vi "Modbus Test Setup.vi"(6 "Mannequin Data":u16[](array[numeric]), 8 "error in (no error)":errorcluster, 10 "Select test case":i32(listbox), 11 "Queue in":refnum<queue>) -> (0 "error out":errorcluster, 3 "Queue out":refnum<queue>)   [LabVIEW 2023]
uses:
  Message Queue/Message Cluster.ctl
  Message Queue/Enqueue Message (Single).vi
  Message Queue/Message Queue.lvlib
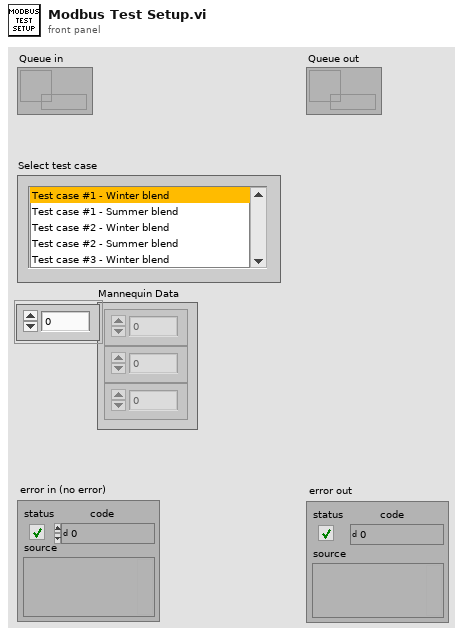
[diagram p1: front panel]
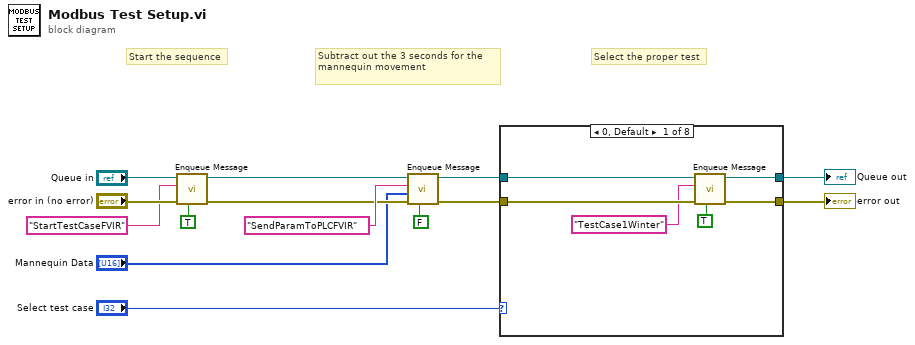
[diagram p0: block diagram]
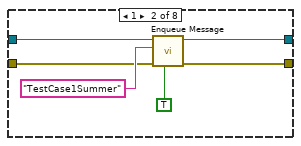
[diagram p2: hidden frame]
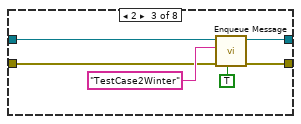
[diagram p3: hidden frame]
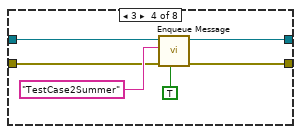
[diagram p4: hidden frame]
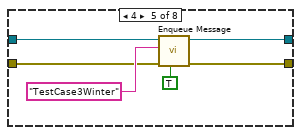
[diagram p5: hidden frame]
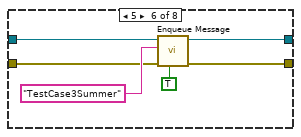
[diagram p6: hidden frame]
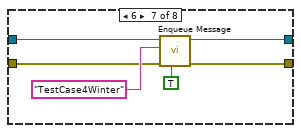
[diagram p7: hidden frame]
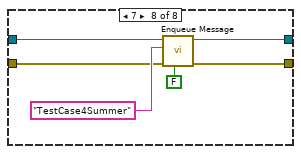
[diagram p8: hidden frame]
diagram:
  # "Select the proper test"
  # "Start the sequence"
  # "Subtract out the 3 seconds for the \nmannequin movement"
  n1 = call-poly "Enqueue Message.vi"("Priority Message? (F)"=TRUE, "error in (no error)"="error in (no error)", "Message"="StartTestCaseFVIR", "Message Queue"="Queue in") -> ("error out"=w2:errorcluster, "dup Message Queue"=w5:refnum<queue>)  [unwired: 6 in]
  n2 = call-poly "Enqueue Message.vi"("Priority Message? (F)"=FALSE, "error in (no error)"=w2, "Message Data"="Mannequin Data", "Message"="SendParamToPLCFVIR", "Message Queue"=w5) -> ("error out"=w3:errorcluster, "dup Message Queue"=w4:refnum<queue>)  [unwired: 5 in]
  n3 = case shown="0, Default" "Select test case" {
    tunnel: w4 -> [w20 w25 w31 w37 w43 w50 w55 w61]
    tunnel: [w17 w24 w30 w36 w42 w49 w54 w60] -> w9
    tunnel: [w19 w23 w29 w35 w41 w48 w53 w59] -> w8
    tunnel: w3 -> [w18 w21 w27 w33 w39 w45 w51 w57]
    frame 0, Default {
      n4 = call-poly "Enqueue Message.vi"("Priority Message? (F)"=TRUE, "error in (no error)"=w18, "Message"="TestCase1Winter", "Message Queue"=w20) -> ("error out"=w17:errorcluster, "dup Message Queue"=w19:refnum<queue>)  [unwired: 6 in]
    }
    frame 1 {
      n5 = call-poly "Enqueue Message.vi"("Priority Message? (F)"=TRUE, "error in (no error)"=w21, "Message"="TestCase1Summer", "Message Queue"=w25) -> ("error out"=w24:errorcluster, "dup Message Queue"=w23:refnum<queue>)  [unwired: 6 in]
    }
    frame 2 {
      n6 = call-poly "Enqueue Message.vi"("Priority Message? (F)"=TRUE, "error in (no error)"=w27, "Message"="TestCase2Winter", "Message Queue"=w31) -> ("error out"=w30:errorcluster, "dup Message Queue"=w29:refnum<queue>)  [unwired: 6 in]
    }
    frame 3 {
      n7 = call-poly "Enqueue Message.vi"("Priority Message? (F)"=TRUE, "error in (no error)"=w33, "Message"="TestCase2Summer", "Message Queue"=w37) -> ("error out"=w36:errorcluster, "dup Message Queue"=w35:refnum<queue>)  [unwired: 6 in]
    }
    frame 4 {
      n8 = call-poly "Enqueue Message.vi"("Priority Message? (F)"=TRUE, "error in (no error)"=w39, "Message"="TestCase3Winter", "Message Queue"=w43) -> ("error out"=w42:errorcluster, "dup Message Queue"=w41:refnum<queue>)  [unwired: 6 in]
    }
    frame 5 {
      n9 = call-poly "Enqueue Message.vi"("Priority Message? (F)"=TRUE, "error in (no error)"=w45, "Message"="TestCase3Summer", "Message Queue"=w50) -> ("error out"=w49:errorcluster, "dup Message Queue"=w48:refnum<queue>)  [unwired: 6 in]
    }
    frame 6 {
      n10 = call-poly "Enqueue Message.vi"("Priority Message? (F)"=TRUE, "error in (no error)"=w51, "Message"="TestCase4Winter", "Message Queue"=w55) -> ("error out"=w54:errorcluster, "dup Message Queue"=w53:refnum<queue>)  [unwired: 6 in]
    }
    frame 7 {
      n11 = call-poly "Enqueue Message.vi"("Priority Message? (F)"=FALSE, "error in (no error)"=w57, "Message"="TestCase4Summer", "Message Queue"=w61) -> ("error out"=w60:errorcluster, "dup Message Queue"=w59:refnum<queue>)  [unwired: 6 in]
    }
  }
  "Queue out" <- w8
  "error out" <- w9
